vi "Dequeue Command.vi"(8 "error in (no error)":errorcluster, 11 "Command Processor Actor in":refnum<class "Command Processor Actor.lvclass">) -> (0 "error out":errorcluster, 2 "Command":refnum<class "Command Actor.lvclass">, 3 "Command Processor Actor out":refnum<class "Command Processor Actor.lvclass">)   [LabVIEW 2014, in "Robot Actor Framework.lvlib" / "Command Processor Actor.lvlib" / "Command Processor Actor.lvclass"]
uses:
  Command Processor Actor.lvclass
  Command Actor/Command Actor Class/Command Actor.lvclass
  Command Processor Actor.lvclass/Command Processor Actor.ctl
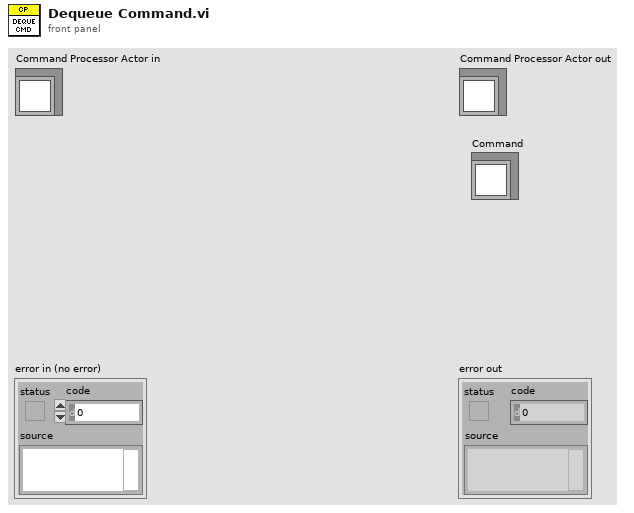
[diagram p1: front panel]
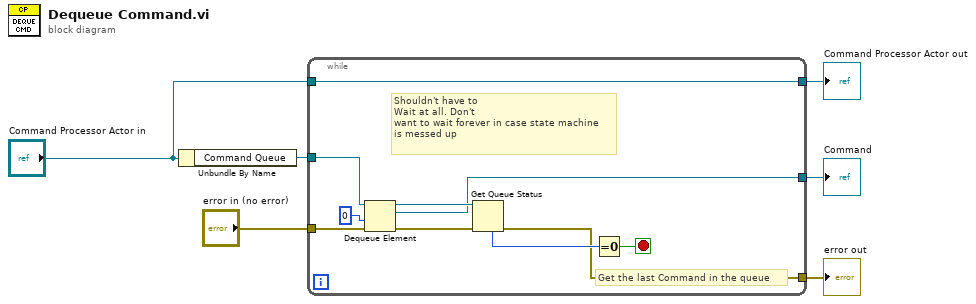
[diagram p0: block diagram]
diagram:
  n1 = Unbundle By Name("Command Processor Actor in") -> ("Command Queue"=w4:refnum<queue>)
  n2 = while {
    tunnel: w4 -> [w16]
    tunnel: [w8] -> w3
    tunnel: "Command Processor Actor in" -> [w9]
    tunnel: [w9] -> w5
    tunnel: "error in (no error)" -> [w11]
    tunnel: [w7] -> w1
    stop <- w14 stop-if-true
    # "Shouldn't have to \nWait at all. Don't\nwant to wait forever in case state machine\nis messed up"
    # "Get the last Command in the queue"
    n3 = Dequeue Element(queue=w16, timeout in ms (-1)=0, error in (no error)=w11) -> (queue out=w15:refnum<queue>, element=w8:refnum<class "Command Actor.lvclass">, error out=w10:errorcluster)  [unwired: 1 out]
    n4 = Get Queue Status(queue=w15, error in (no error)=w10) -> (error out=w7:errorcluster, # elements in queue=w13:i32)  [unwired: 1 in, 6 out]
    n5 = Equal To 0?(x=w13) -> (x = 0?=w14:bool)
  }
  "error out" <- w1
  "Command Processor Actor out" <- w5
  "Command" <- w3
